vi "GUI_HTU_Visa.vi"() -> ()   [LabVIEW 2020]
uses:
  Shared/GUI_Template/GUI_master/tcp_new_data_event.ctl
  Shared/GUI_Template/GUI_master/tcp new data cluster.ctl
panel:
  in  "AnalogOutput.Channel 15::1":dbl caption="ao15" min=-10.0 max=10.0 format="%.3f"
  in  "AnalogOutput.Channel 14::1":dbl caption="ao14" min=-10.0 max=10.0 format="%.3f"
  in  "AnalogOutput.Channel 13::1":dbl caption="ao13" min=-10.0 max=10.0 format="%.3f"
  in  "AnalogOutput.Channel 12::1":dbl caption="ao12" min=-10.0 max=10.0 format="%.3f"
  in  "AnalogOutput.Channel 11::1":dbl caption="ao11" min=-10.0 max=10.0 format="%.3f"
  in  "AnalogOutput.Channel 10::1":dbl caption="ao10" min=-10.0 max=10.0 format="%.3f"
  in  "AnalogOutput.Channel 9::1":dbl caption="ao9" min=-10.0 max=10.0 format="%.3f"
  in  "AnalogOutput.Channel 8::1":dbl caption="o8" min=-10.0 max=10.0 format="%.3f"
  out "AI_mean.Channel 23::2":dbl caption="ai23" min=0.0 max=0.0 format="%.3f"
  out "AI_mean.Channel 22::2":dbl caption="ai22" min=0.0 max=0.0 format="%.3f"
  out "AI_mean.Channel 21::2":dbl caption="ai21" min=0.0 max=0.0 format="%.3f"
  out "AI_mean.Channel 20::2":dbl caption="ai20" min=0.0 max=0.0 format="%.3f"
  out "AI_mean.Channel 19::2":dbl caption="ai19" min=0.0 max=0.0 format="%.3f"
  out "AI_mean.Channel 18::2":dbl caption="ai18" min=0.0 max=0.0 format="%.3f"
  out "AI_mean.Channel 17::2":dbl caption="ai17" min=0.0 max=0.0 format="%.3f"
  out "AI_mean.Channel 16::2":dbl caption="ai16" min=0.0 max=0.0 format="%.3f"
  in  "AnalogOutput.Channel 7::1":dbl caption="ao7" min=-10.0 max=10.0 format="%.3f"
  in  "AnalogOutput.Channel 6::1":dbl caption="ao6" min=-10.0 max=10.0 format="%.3f"
  in  "AnalogOutput.Channel 5::1":dbl caption="ao5" min=-10.0 max=10.0 format="%.3f"
  in  "AnalogOutput.Channel 4::1":dbl caption="ao4" min=-10.0 max=10.0 format="%.3f"
  in  "AnalogOutput.Channel 3::1":dbl caption="ao3" min=-10.0 max=10.0 format="%.3f"
  in  "AnalogOutput.Channel 2::1":dbl caption="ao2" min=-10.0 max=10.0 format="%.3f"
  in  "AnalogOutput.Channel 1::1":dbl caption="ao1" min=-10.0 max=10.0 format="%.3f"
  in  "AnalogOutput.Channel 0::1":dbl caption="ao0" min=-10.0 max=10.0 format="%.3f"
  out "AI_mean.Channel 7::2":dbl caption="ai7" min=0.0 max=0.0 format="%.3f"
  out "AI_mean.Channel 6::2":dbl caption="ai6" min=0.0 max=0.0 format="%.3f"
  out "AI_mean.Channel 5::2":dbl caption="ai5" min=0.0 max=0.0 format="%.3f"
  out "AI_mean.Channel 4::2":dbl caption="ai4" min=0.0 max=0.0 format="%.3f"
  out "AI_mean.Channel 3::2":dbl caption="ai3" min=0.0 max=0.0 format="%.3f"
  out "AI_mean.Channel 2::2":dbl caption="ai2" min=0.0 max=0.0 format="%.3f"
  out "AI_mean.Channel 1::2":dbl caption="ai1" min=0.0 max=0.0 format="%.3f"
  in  "GUIdevice 3":string="U_VisaPlungers"
  out "AI_mean.Channel 0::2":dbl caption="ai0" min=0.0 max=0.0 format="%.3f"
  in  "UDP error message":string
  in  "GUIdevice 2":string="U_VisaMagReadback"
  in  "GUIdevice 1":string="U_VisaMagControl"
  out "error IO 2":errorcluster
  out "tcp data event":T1
  in  "stop":bool
  # "Visa steering"
  # "V1V"
  # "V2H"
  # "V2V"
  # "V3H"
  # "V3V"
  # "V4H"
  # "V4V"
  # "V1H"
  # "Command"
  # "readback"
  # "V5V"
  # "V6H"
  # "V6V"
  # "V7H"
  # "V7V"
  # "V8H"
  # "V8V"
  # "V5H"
  # "Command"
  # "readback"
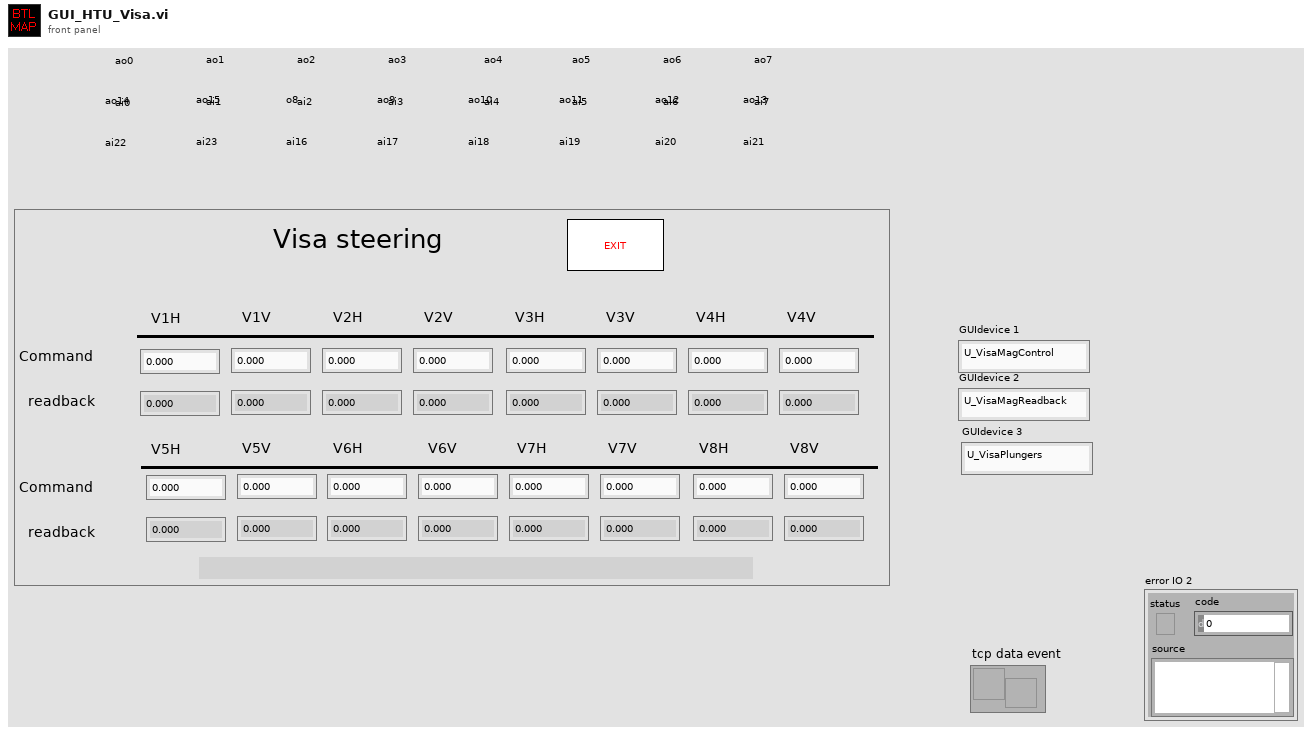
[diagram p1: front panel]
types:
  T1 = typedef "tcp_new_data_event.ctl" = refnum<user-event>
  T2 = typedef "tcp new data cluster.ctl" = cluster{"EventEnum":enum16{"new data", "connection status update"}, "Device name":string}
  T3 = enum32{"invalid app kind", "Development System", "Run Time System", "Student Edition", "Embedded LabVIEW", "Evaluation", "Custom"}
  T4 = enum32{"Invalid", "Standard", "Closed", "Hidden", "Minimized", "Maximized"}
  T5 = cluster{"Core":cluster{"Current VI Reference":refnum<vi>, "Close Panel on Exit?":bool}, "CurrentGraph1":dbl[][], "EMQ1PolaritySwitched":bool, "EMQ2PolaritySwitched":bool, "EMQ3PolaritySwitched":bool, "DegaussEMQ1":bool, "degauss loop":i32, "EMQ1DegaussSetCur":dbl, "EMQ2DegaussSetCur":dbl, "EMQ3DegaussSetCur":dbl, "last chart update tck":i32}
  T6 = cluster{"Current VI Reference":refnum<vi>, "Close Panel on Exit?":bool}
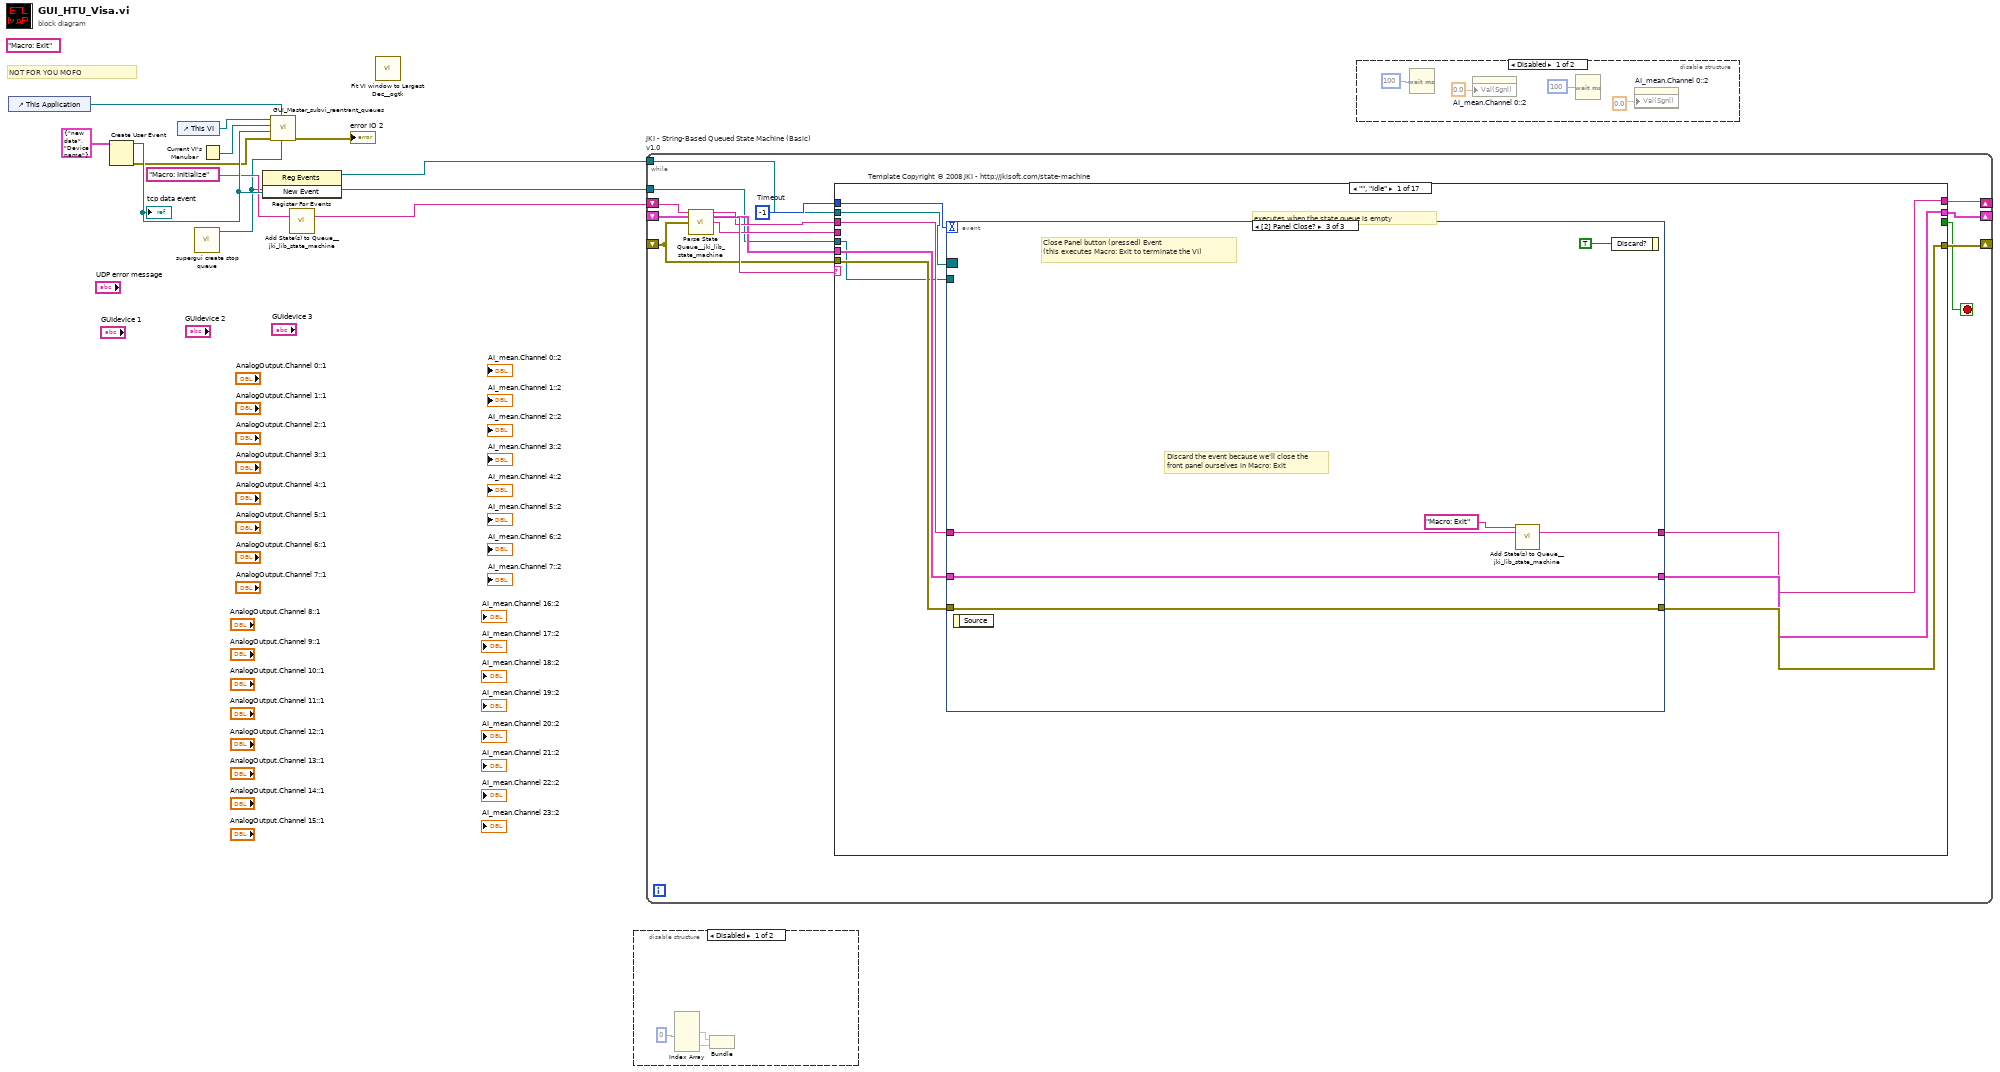
[diagram p0: block diagram]
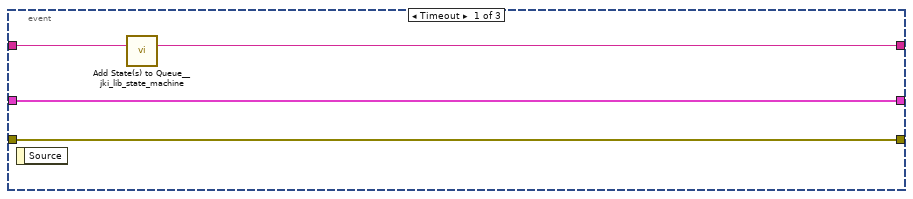
[diagram p4: hidden frame]
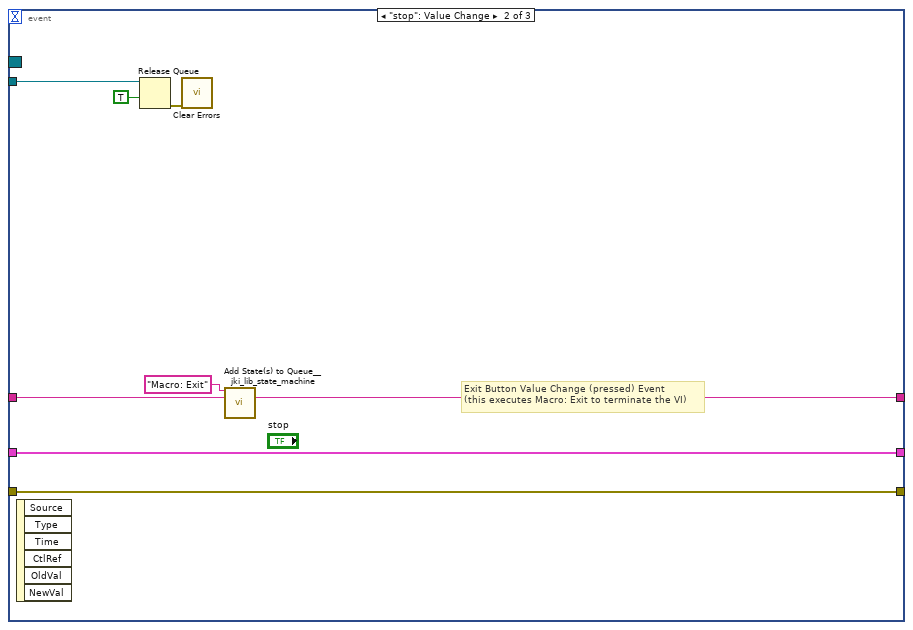
[diagram p5: hidden frame]
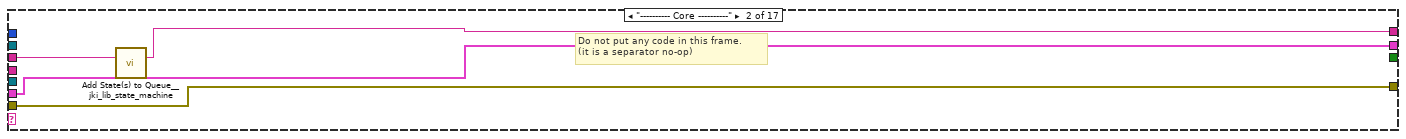
[diagram p6: hidden frame]
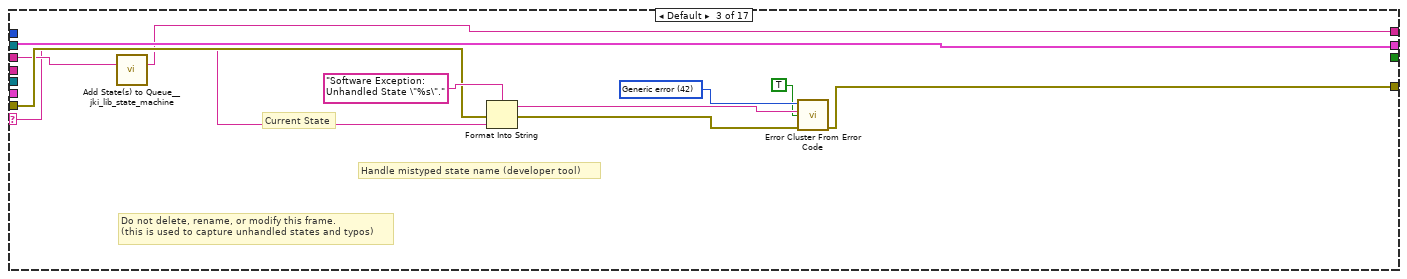
[diagram p7: hidden frame]
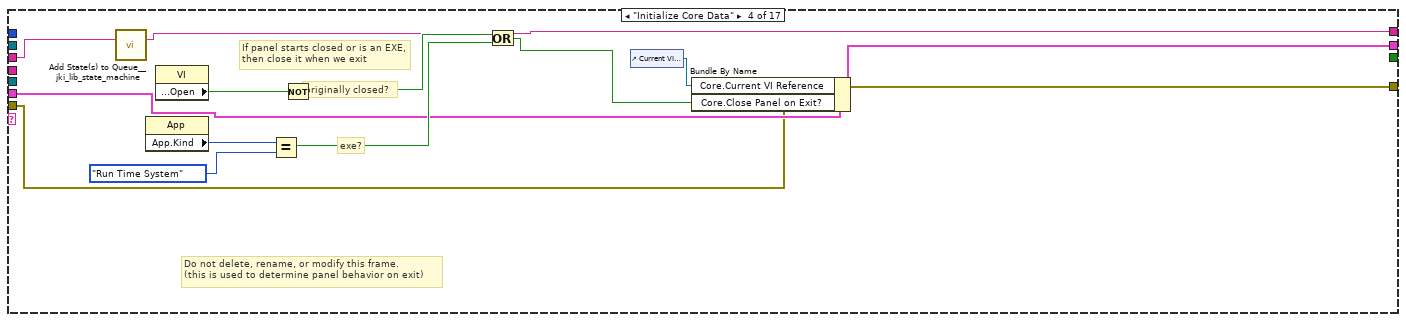
[diagram p8: hidden frame]
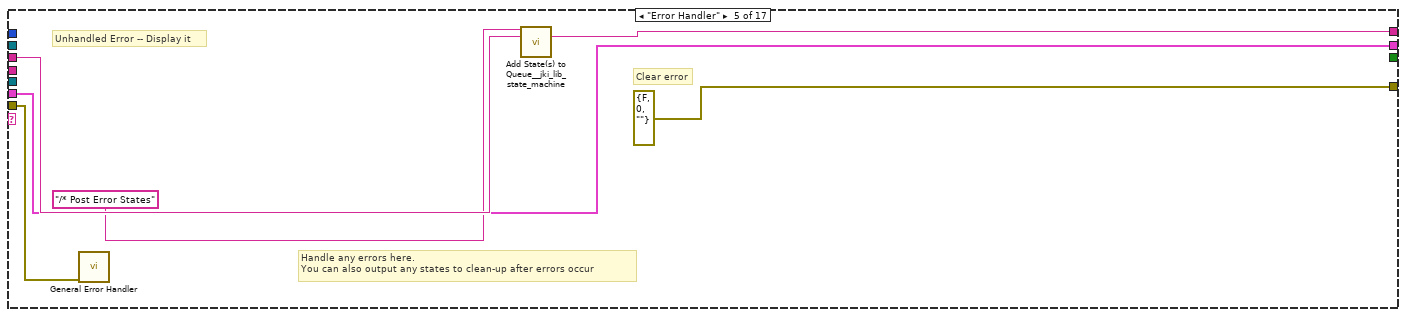
[diagram p9: hidden frame]
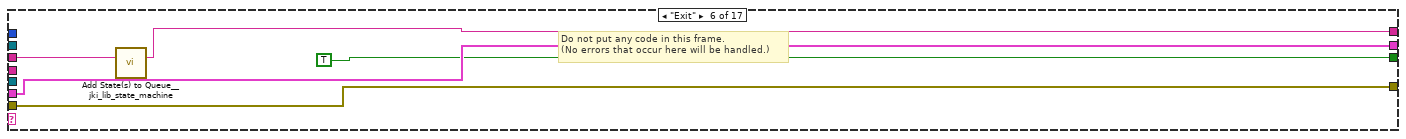
[diagram p10: hidden frame]
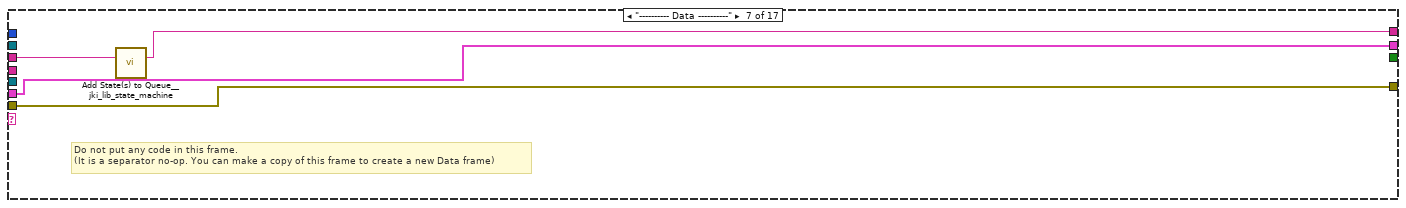
[diagram p11: hidden frame]
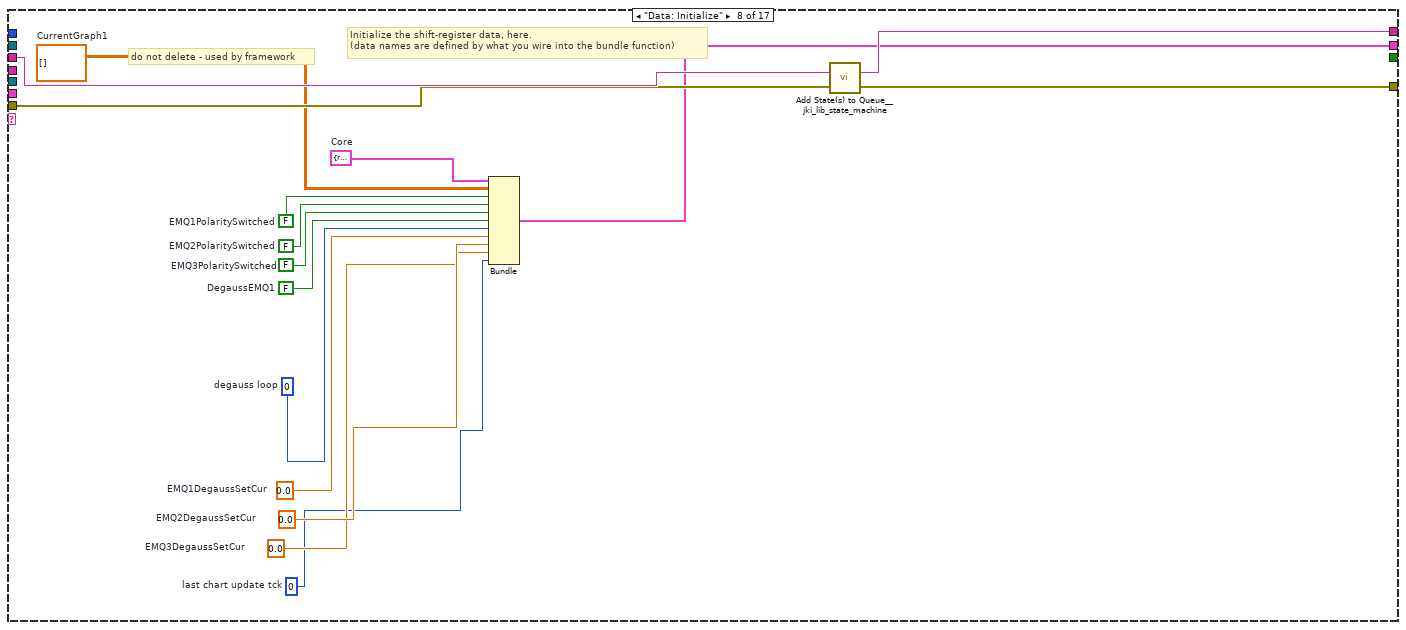
[diagram p12: hidden frame]
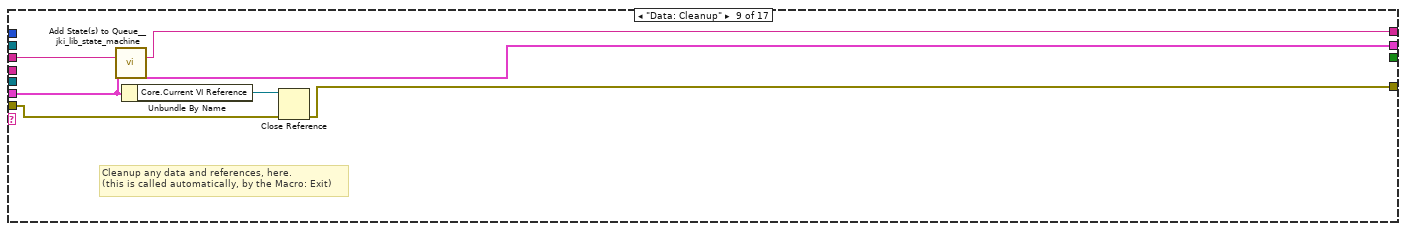
[diagram p13: hidden frame]
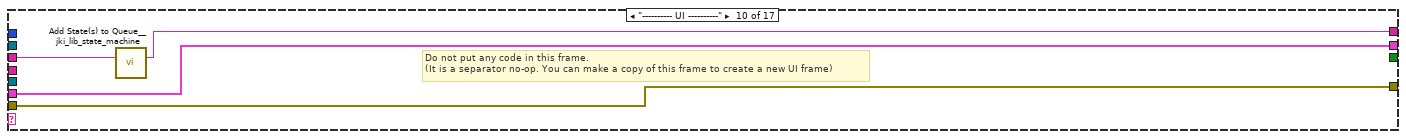
[diagram p14: hidden frame]
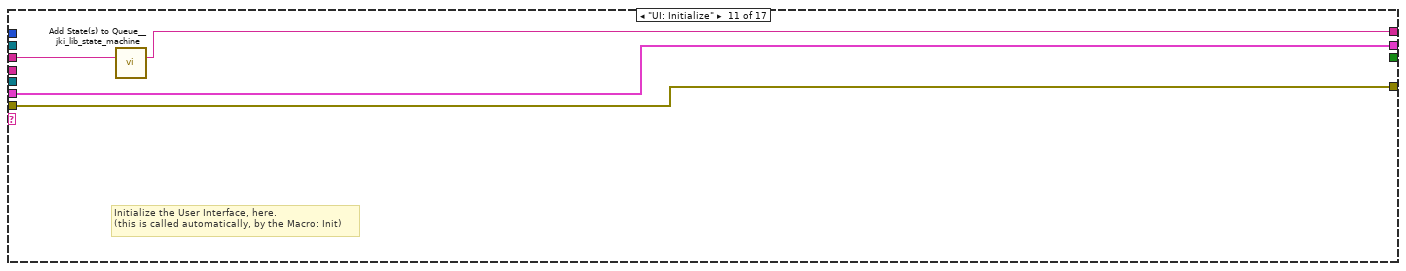
[diagram p15: hidden frame]
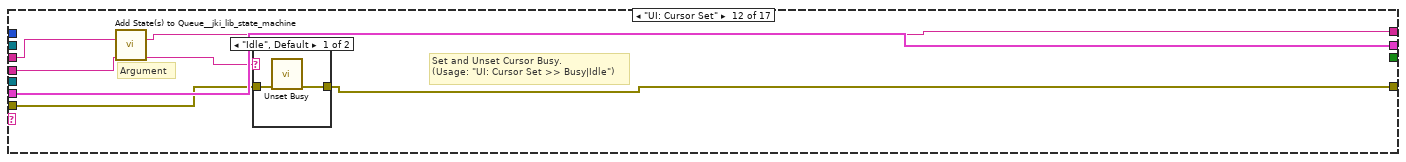
[diagram p16: hidden frame]
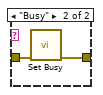
[diagram p17: hidden frame]
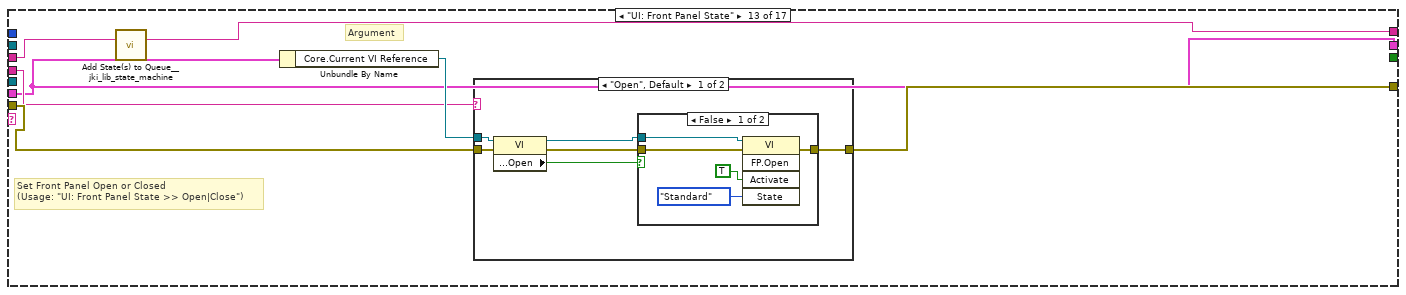
[diagram p18: hidden frame]
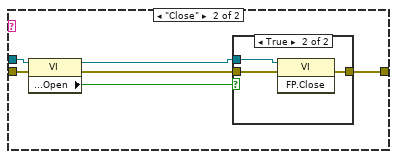
[diagram p20: hidden frame]
diagram:
  (unwired) "Macro: Exit"
  # "NOT FOR YOU MOFO"
  n1 = control-ref of="This Application"() -> (w11:refnum<vi>)
  n2 = Create User Event(user event datatype=T2 {"EventEnum"=enum."new data", "Device name"="Device name"} ("New Event")) -> (user event=w10:refnum<user-event>, error out=w9:errorcluster)  [unwired: 1 in]
  "tcp data event" <- w10
  n3 = control-ref of="This VI"() -> (w5:refnum<vi>)
  n4 = call "supergui create stop queue.vi"() -> ("STOP Queue out"=w1:refnum<queue>)  [unwired: 11 in]
  n5 = Current VI's Menubar() -> (w7:refnum<k9>)
  n6 = register-events(w10) -> (reference out=w2:refnum<event-registration>)  [unwired: 2 in, 1 out]
  n7 = call "GUI_Master_subvi_reentrant_queues.vi"("STOP Queue in"=w1, "This Application"=w11, "error in (no error)"=w9, "tcp data event"=w10, "Caller menu reference"=w7, "Caller VI ref"=w5) -> ("error out"=→"error IO 2":errorcluster)  [unwired: 5 in]
  n8 = call <vilib>:"Add State(s) to Queue__jki_lib_state_machine.vi"("State(s) in (\"\")"="Macro: Initialize") -> ("States Out"=w3:string)  [unwired: 14 in]
  n9 = call <userlib>:"Fit VI window to Largest Dec__ogtk.vi"() -> ()  [unwired: 6 in, 2 out]
  n10 = disable-structure shown="Disabled" {
    frame Disabled {
      n11 = Index Array(index (col) #1=0 ("disabled index (col)")) -> (array=w16:dbl[][], element #1=w12, element #2=w13)  [unwired: 3 in]
      n12 = Bundle(w12, w13) -> (w14:cluster{void, void})  [unwired: 1 in]
    }
    frame Enabled {
    }
  }
  n13 = while "JKI - String-Based Queued State Machine (Basic) v1.0" {
    shift-right: [w23] -> _
    shift-left: _ -> [w22]
    shift-right: [w25] -> _
    shift-left: _ -> [w20]
    shift-right: [w17] -> _
    shift-left: w3 -> [w26]
    tunnel: w2 -> [w19]
    tunnel: w1 -> [w18]
    stop <- w24 stop-if-true
    w21 = -1  # Timeout
    # "Template Copyright © 2008 JKI - http://jkisoft.com/state-machine"
    n14 = call <vilib>:"Parse State Queue__jki_lib_state_machine.vi"("State Queue"=w26, "Error In (no error)"=w20) -> ("Remaining States"=w28:string, "Current State"=w29:string, "Arguments"=w27:string)  [unwired: 11 in]
    n15 = case shown="\"\", \"Idle\"" w29 {
      selector: w29 -> [_ _ w62 _ _ _ _ _ _ _ _ _ _ _ _ _ _]
      tunnel: w28 -> [w38 w60 w65 w83 w89 w94 w98 w113 w119 w123 w127 w133 w144 w170 w175 w185 w189]
      tunnel: w27 -> [_ _ _ _ _ _ _ _ _ _ _ w129 w140 _ _ _ _]
      tunnel: w22 -> [w37 w58 w64 w75 w88 w93 w96 _ w115 w121 w126 w132 w139 w168 w173 w177 w187]
      tunnel: [w36 w59 w67 w72 errorcluster {"status"=FALSE, "code"=0, "source"=""} ("error out") w92 w97 w112 w117 w122 w125 w130 w142 w169 w174 w184 w188] -> w25
      tunnel: w20 -> [w35 w59 w66 w72 w87 w92 w97 w112 w118 w122 w125 w131 w143 w169 w174 w184 w188]
      tunnel: [_ _ _ _ _ TRUE _ _ _ _ _ _ _ _ _ _ _] -> w24
      tunnel: [w32 w58 w64 w74 w88 w93 w96 w102 w115 w121 w126 w132 w139 w168 w173 w177 w187] -> w23
      tunnel: w21 -> [w34 _ _ _ _ _ _ _ _ _ _ _ _ _ _ _ _]
      tunnel: w19 -> [w30 _ _ _ _ _ _ _ _ _ _ _ _ _ _ _ _]
      tunnel: w18 -> [w33 _ _ _ _ _ _ _ _ _ _ _ _ _ _ _ _]
      tunnel: [w31 w57 w61 w73 w84 w90 w95 w108 w114 w120 w124 w128 w138 w167 w171 w176 w186] -> w17
      frame "", "Idle" {
        # "executes when the state queue is empty"
        n16 = event shown="[2] Panel Close?" {
          selector: w30 -> [_ _ _]
          dyn-events: _ -> [_ _ _]
          timeout: w34 -> [_ _ _]
          tunnel: w38 -> [w42 w50 w56]
          tunnel: [w41 w49 w55] -> w31
          tunnel: w37 -> [w39 w47 w53]
          tunnel: [w40 w48 w54] -> w36
          tunnel: w35 -> [w40 w48 w54]
          tunnel: [w39 w47 w53] -> w32
          tunnel: w33 -> [_ w44 _]
          event Timeout {
            n17 = event-data() -> ()  [unwired: 1 in, 1 out]
            n18 = call <vilib>:"Add State(s) to Queue__jki_lib_state_machine.vi"("State(s) in (\"\")"=w42) -> ("States Out"=w41:string)  [unwired: 14 in]
          }
          event "stop": Value Change {
            # "Exit Button Value Change (pressed) Event\n(this executes Macro: Exit to terminate the VI)"
            n19 = event-data() -> ()  [unwired: 1 in, 6 out]
            n20 = Release Queue(queue=w44, force destroy? (F)=TRUE) -> (error out=w45:errorcluster)  [unwired: 1 in, 2 out]
            n21 = call <vilib>:"Clear Errors.vi"("error in (no error)"=w45) -> ()  [unwired: 5 in, 2 out]
            n22 = call <vilib>:"Add State(s) to Queue__jki_lib_state_machine.vi"("State(s) in Front (\"\")"="Macro: Exit", "State(s) in (\"\")"=w50) -> ("States Out"=w49:string)  [unwired: 13 in]
          }
          event Panel Close? {
            # "Discard the event because we'll close the front panel ourselves in Macro: Exit"
            # "Close Panel button (pressed) Event\n(this executes Macro: Exit to terminate the VI)"
            n23 = event-data() -> ()  [unwired: 1 in, 1 out]
            n24 = call <vilib>:"Add State(s) to Queue__jki_lib_state_machine.vi"("State(s) in Front (\"\")"="Macro: Exit", "State(s) in (\"\")"=w56) -> ("States Out"=w55:string)  [unwired: 13 in]
            n25 = event-data("Discard?"=TRUE) -> ()  [unwired: 1 in, 1 out]
          }
        }
      }
      frame "---------- Core ----------" {
        # "Do not put any code in this frame.\n(it is a separator no-op)"
        n26 = call <vilib>:"Add State(s) to Queue__jki_lib_state_machine.vi"("State(s) in (\"\")"=w60) -> ("States Out"=w57:string)  [unwired: 14 in]
      }
      frame Default {
        w70 = 42 items=["No error", "Argument error", "Memory is full", "Out of zone", "End of file", "File already open", "Generic file I/O error", "File not found", "File permission error", "Disk is full", "Duplicate path", "Too many files open", "System feature not enabled", "Resource file not found", "Cannot add resource", "Resource not found", "Image not found", "Image memory error", "Pen does not exist", "Config type invalid", "Config token not found", "Config parse error", "Config memory error", "Bad external code format", "Bad external code offset", "External code not present", "Null window", "Destroy window error", "Null menu", "Print aborted", "Bad print record", "Print driver error", "Windows error during printing", "Memory error during printing", "Print dialog error", "Generic print error", "Invalid device refnum", "Device not found", "Device parameter error", "Device unit error", "Cannot open device", "Device call aborted", "Generic error", "Cancelled by user", "Object ID too low", "Object ID too high", "Object not in heap", "Unknown heap", "Unknown object (invalid DefProc)", "Unknown object (DefProc not in table)", "Message out of range", "Invalid (null) method", "Unknown message", "Manager call not supported", "Bad address", "Network operation in progress", "Network operation timed out", "Connection is busy", "Network attribute not supported", "Network error", "Address in use", "System out of memory", "Connection aborted", "Connection refused", "Not connected", "Already connected", "Connection closed", "Initialization error (interapplication manager)", "Bad occurrence", "Wait on unbound occurrence handler", "Occurrence queue overflow", "Datalog type conflict", "Unused", "Unrecognized type (interapplication manager)", "Memory corrupt", "Failed to make temporary DLL", "Old CIN version", "Drag socket not found", "Failed to load drop-object", "Failed to register OLE object", "Failed to release OLE object", "Format specifier type mismatch", "Unknown format specifier", "Too few format specifiers", "Too many format specifiers", "Scan failed", "Newer CIN version", "Error converting to variant", "Runtime menu error", "Password tampered", "Variant attribute not found", "Incompatible variant data type", "Event data is not available", "Event Store is not present", "Occurrence is not found", "Event Queue is not created", "Event info is not available", "Refnum passed is NULL", "Error retrieving Class GUID", "Error retrieving CoClass GUID", "Error retrieving TypeLib GUID.", "Bad built application magic bytes.", "Specific driver is different from the specific driver associated with the Logical Name.", "There is no session opened to the class driver.", "Max Error", "MAX - Error with config objects", "MAX - Error loading configuration", "MAX - Group not supported"]
        # "Current State"
        # "Do not delete, rename, or modify this frame.\n(this is used to capture unhandled states and typos)"
        # "Handle mistyped state name (developer tool)"
        n27 = call <vilib>:"Add State(s) to Queue__jki_lib_state_machine.vi"("State(s) in (\"\")"=w65) -> ("States Out"=w61:string)  [unwired: 14 in]
        n28 = Format Into String(format string="Software Exception: Unhandled State \"%s\"." ("message"), error in=w66, w62) -> (resulting string=w69:string, error out=w68:errorcluster)  [unwired: 1 in]
        n29 = call <vilib>:"Error Cluster From Error Code.vi"("show call chain? (False)"=TRUE, "error in (no error)"=w68, "error message (\"\")"=w69, "error code (0)"=w70) -> ("error out"=w67:errorcluster)  [unwired: 5 in]
      }
      frame "Initialize Core Data" {
        # "Do not delete, rename, or modify this frame.\n(this is used to determine panel behavior on exit)"
        # "originally closed?"
        # "exe?"
        # "If panel starts closed or is an EXE, then close it when we exit"
        n30 = call <vilib>:"Add State(s) to Queue__jki_lib_state_machine.vi"("State(s) in (\"\")"=w83) -> ("States Out"=w73:string)  [unwired: 14 in]
        n31 = property class="App"() -> ("App.Kind"=w81:T3)  [unwired: 2 in, 2 out]
        n32 = property class="VI"() -> ("Front Panel.Open"=w82:bool)  [unwired: 2 in, 2 out]
        n33 = Equal?(x=w81, y=T3."Run Time System" ("Application:Kind")) -> (x = y?=w78:bool)
        n34 = Not(x=w82) -> (.not. x?=w79:bool)
        n35 = Or(x=w79, y=w78) -> (x .or. y?=w77:bool)
        n36 = control-ref of="Current VI Reference"() -> (w76:refnum<vi>)
        n37 = Bundle By Name(cluster=w75, "Core.Current VI Reference"=w76, "Core.Close Panel on Exit?"=w77) -> (w74:T5)
      }
      frame "Error Handler" {
        # "Unhandled Error -- Display it"
        # "Handle any errors here.\nYou can also output any states to clean-up after errors occur"
        # "Clear error"
        n38 = call <vilib>:"General Error Handler.vi"("error in (no error)"=w87) -> ()  [unwired: 10 in, 5 out]
        n39 = call <vilib>:"Add State(s) to Queue__jki_lib_state_machine.vi"("State(s) in Front (\"\")"="/* Post Error States", "State(s) in (\"\")"=w89) -> ("States Out"=w84:string)  [unwired: 13 in]
      }
      frame "Exit" {
        # "Do not put any code in this frame.\n(No errors that occur here will be handled.)"
        n40 = call <vilib>:"Add State(s) to Queue__jki_lib_state_machine.vi"("State(s) in (\"\")"=w94) -> ("States Out"=w90:string)  [unwired: 14 in]
      }
      frame "---------- Data ----------" {
        # "Do not put any code in this frame.\n(It is a separator no-op. You can make a copy of this frame to create a new Data frame)"
        n41 = call <vilib>:"Add State(s) to Queue__jki_lib_state_machine.vi"("State(s) in (\"\")"=w98) -> ("States Out"=w95:string)  [unwired: 14 in]
      }
      frame "Data: Initialize" {
        w99 = 0  # last chart update tck
        w100 = 0.0  # EMQ3DegaussSetCur
        w101 = 0.0  # EMQ2DegaussSetCur
        w103 = 0.0  # EMQ1DegaussSetCur
        w104 = 0  # degauss loop
        w105 = FALSE  # DegaussEMQ1
        w106 = FALSE  # EMQ3PolaritySwitched
        w107 = FALSE  # EMQ2PolaritySwitched
        w109 = FALSE  # EMQ1PolaritySwitched
        w110 = dbl[][] []  # CurrentGraph1
        w111 = T6 {"Current VI Reference"=refnum, "Close Panel on Exit?"=FALSE}  # Core
        # "do not delete - used by framework"
        # "Initialize the shift-register data, here.\n(data names are defined by what you wire into the bundle function)"
        n42 = Bundle("Core"=w111, "CurrentGraph1"=w110, "EMQ1PolaritySwitched"=w109, "EMQ2PolaritySwitched"=w107, "EMQ3PolaritySwitched"=w106, "DegaussEMQ1"=w105, "degauss loop"=w104, "EMQ1DegaussSetCur"=w103, "EMQ2DegaussSetCur"=w101, "EMQ3DegaussSetCur"=w100, "last chart update tck"=w99) -> (w102:T5)  [unwired: 1 in]
        n43 = call <vilib>:"Add State(s) to Queue__jki_lib_state_machine.vi"("State(s) in (\"\")"=w113) -> ("States Out"=w108:string)  [unwired: 14 in]
      }
      frame "Data: Cleanup" {
        # "Cleanup any data and references, here.\n(this is called automatically, by the Macro: Exit)"
        n44 = call <vilib>:"Add State(s) to Queue__jki_lib_state_machine.vi"("State(s) in (\"\")"=w119) -> ("States Out"=w114:string)  [unwired: 14 in]
        n45 = Unbundle By Name(w115) -> ("Core.Current VI Reference"=w116:refnum<vi>)
        n46 = Close Reference(reference=w116, error in (no error)=w118) -> (error out=w117:errorcluster)
      }
      frame "---------- UI ----------" {
        # "Do not put any code in this frame.\n(It is a separator no-op. You can make a copy of this frame to create a new UI frame)"
        n47 = call <vilib>:"Add State(s) to Queue__jki_lib_state_machine.vi"("State(s) in (\"\")"=w123) -> ("States Out"=w120:string)  [unwired: 14 in]
      }
      frame "UI: Initialize" {
        # "Initialize the User Interface, here.\n(this is called automatically, by the Macro: Init)"
        n48 = call <vilib>:"Add State(s) to Queue__jki_lib_state_machine.vi"("State(s) in (\"\")"=w127) -> ("States Out"=w124:string)  [unwired: 14 in]
      }
      frame "UI: Cursor Set" {
        # "Argument"
        # "Set and Unset Cursor Busy.\n(Usage: \"UI: Cursor Set >> Busy|Idle\")"
        n49 = call <vilib>:"Add State(s) to Queue__jki_lib_state_machine.vi"("State(s) in (\"\")"=w133) -> ("States Out"=w128:string)  [unwired: 14 in]
        n50 = case shown="\"Idle\", Default" w129 {
          tunnel: w131 -> [w135 w137]
          tunnel: [w134 w136] -> w130
          frame "Idle", Default {
            n51 = call <vilib>:"Unset Busy.vi"("error in (no error)"=w135) -> ("error out"=w134:errorcluster)  [unwired: 10 in]
          }
          frame "Busy" {
            n52 = call <vilib>:"Set Busy.vi"("error in (no error)"=w137) -> ("error out"=w136:errorcluster)  [unwired: 9 in, 1 out]
          }
        }
      }
      frame "UI: Front Panel State" {
        # "Argument"
        # "Set Front Panel Open or Closed\n(Usage: \"UI: Front Panel State >> Open|Close\")"
        n53 = call <vilib>:"Add State(s) to Queue__jki_lib_state_machine.vi"("State(s) in (\"\")"=w144) -> ("States Out"=w138:string)  [unwired: 14 in]
        n54 = Unbundle By Name(w139) -> ("Core.Current VI Reference"=w141:refnum<vi>)
        n55 = case shown="\"Open\", Default" w140 {
          tunnel: w143 -> [w149 w161]
          tunnel: [w150 w162] -> w142
          tunnel: w141 -> [w145 w157]
          frame "Open", Default {
            n56 = property class="VI"(reference=w145, error in=w149) -> (reference out=w147:refnum<vi>, error out=w148:errorcluster, "Front Panel.Open"=w146:bool)
            n57 = case shown="False" w146 {
              tunnel: [w153 w156] -> w150
              tunnel: w148 -> [w152 w156]
              tunnel: w147 -> [w151 _]
              frame False {
                n58 = invoke class="VI" method="FP.Open"(reference=w151, error in=w152, "Activate"=TRUE, "State"=T4."Standard") -> (error out=w153:errorcluster)  [unwired: 1 in, 4 out]
              }
              frame True {
              }
            }
          }
          frame "Close" {
            n59 = property class="VI"(reference=w157, error in=w161) -> (reference out=w159:refnum<vi>, error out=w160:errorcluster, "Front Panel.Open"=w158:bool)
            n60 = case shown="True" w158 {
              tunnel: [w163 w166] -> w162
              tunnel: w160 -> [w163 w165]
              tunnel: w159 -> [_ w164]
              frame False {
              }
              frame True {
                n61 = invoke class="VI" method="FP.Close"(reference=w164, error in=w165) -> (error out=w166:errorcluster)  [unwired: 1 in, 2 out]
              }
            }
          }
        }
      }
      frame "---------- Macro ----------" {
        # "Do not put any code in this frame.\n(It is a separator no-op. You can make a copy of this frame to create a new Macro frame)"
        n62 = call <vilib>:"Add State(s) to Queue__jki_lib_state_machine.vi"("State(s) in (\"\")"=w170) -> ("States Out"=w167:string)  [unwired: 14 in]
      }
      frame "Macro: Initialize" {
        w172 = "Data: Initialize\nInitialize Core Data\nUI: Initialize\nUI: Front Panel State >> Open"  # Data: Initialize Initialize Core Data UI: Initialize UI: Front Panel State >> Open
        # "Initialization Macro\n(This is called once, when the VI starts)"
        n63 = call <vilib>:"Add State(s) to Queue__jki_lib_state_machine.vi"("State(s) in Front (\"\")"=w172, "State(s) in (\"\")"=w175) -> ("States Out"=w171:string)  [unwired: 13 in]
      }
      frame "Macro: Exit" {
        # "Exit Macro\n(This is called once, when the VI exits)"
        n64 = Unbundle By Name(w177) -> ("Core.Close Panel on Exit?"=w178:bool)
        n65 = Select(t="UI: Front Panel State >> Close", s=w178, f="") -> (s? t:f=w181:string)
        n66 = call <vilib>:"Add State(s) to Queue__jki_lib_state_machine.vi"("State(s) in (\"\")"=w181, "State(s) at Back (\"\")"="Data: Cleanup\nExit") -> ("States Out"=w179:string)  [unwired: 13 in]
        n67 = call <vilib>:"Add State(s) to Queue__jki_lib_state_machine.vi"("State(s) in Front (\"\")"=w179, "State(s) in (\"\")"=w185) -> ("States Out"=w176:string)  [unwired: 13 in]
      }
      frame "---------- New Category ----------" {
        n68 = call <vilib>:"Add State(s) to Queue__jki_lib_state_machine.vi"("State(s) in (\"\")"=w189) -> ("States Out"=w186:string)  [unwired: 14 in]
      }
    }
  }
  n69 = disable-structure shown="Disabled" {
    frame Disabled {
      n70 = Wait (ms)(milliseconds to wait=u32 100) -> ()  [unwired: 1 out]
      n71 = property on="AI_mean.Channel 0::2" class="DigNum (strict)"("Val(Sgnl)"=0.0 ("Value (Signaling)")) -> ()  [unwired: 2 in, 2 out]
      n72 = Wait (ms)(milliseconds to wait=u32 100) -> ()  [unwired: 1 out]
      n73 = property on="AI_mean.Channel 0::2" class="DigNum (strict)"("Val(Sgnl)"=0.0 ("Value (Signaling)")) -> ()  [unwired: 2 in, 2 out]
    }
    frame Enabled {
    }
  }
